vi "UniqueIDs 2 ProfileIDs.vi"(0 "Unique IDs":string[](array[string])) -> (4 "Profile IDs":string[](array[string]))   [LabVIEW 2013]
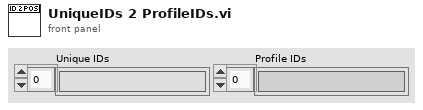
[diagram p1: front panel]
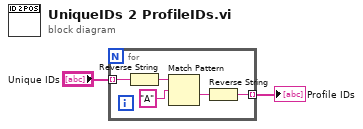
[diagram p0: block diagram]
diagram:
  n1 = for {
    tunnel: "Unique IDs" -> [w7] mode=indexing
    tunnel: [w3] -> w1 mode=indexing
    n2 = Reverse String(1:w7) -> (0:w6:string)
    n3 = Match Pattern(string=w6, regular expression="A") -> (after substring=w4:string)  [unwired: 1 in, 3 out]
    n4 = Reverse String(1:w4) -> (0:w3:string)
  }
  "Profile IDs" <- w1
